vi "Set Periodic Log Filter.vi"(10 "PeriodicLogFilter":T1={"Enable"=TRUE, "Threshold(#/s)"=2.0, "CheckPeriod(s)"=1.0}, 11 "GlobalLogFilter In":refnum<class "LogFilter.lvclass">) -> (3 "GlobalLogFilter Out":refnum<class "LogFilter.lvclass">)   [LabVIEW 2017, in "Communicable State Machine.lvlib" / "LogFilter.lvclass"]
uses:
  LogFilter.lvclass
  LogFilter.lvclass/LogFilter.ctl
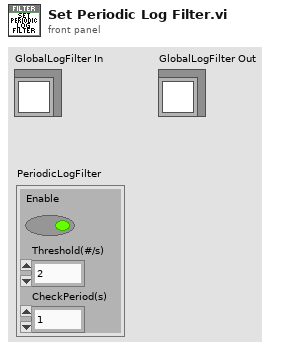
[diagram p1: front panel]
types:
  T1 = cluster{"Enable":bool, "Threshold(#/s)":dbl, "CheckPeriod(s)":dbl}
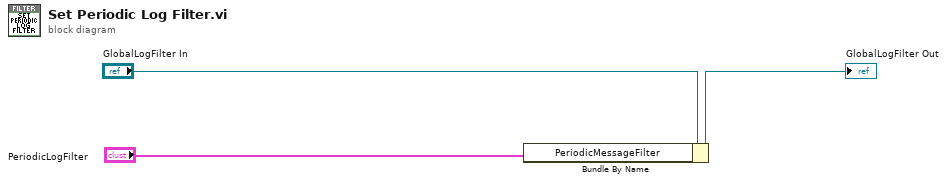
[diagram p0: block diagram]
diagram:
  n1 = Bundle By Name(cluster="GlobalLogFilter In", "PeriodicMessageFilter"="PeriodicLogFilter") -> (→"GlobalLogFilter Out":refnum<class "LogFilter.lvclass">)
